vi "MRC Ds Comms Wait For System Server.vi"(8 "error in (no error)":errorcluster, 11 "waitTimeMs":u32) -> (0 "error out":errorcluster)   [LabVIEW 2026, in "MrcLib.lvlib"]
doc: "MRC_Bool MRC_CALLCONV MRC_DsComms_WaitForSystemServer(uint32_t waitTimeMs);"
uses:
  MrcLib.lvlib
  MrcLib.dll
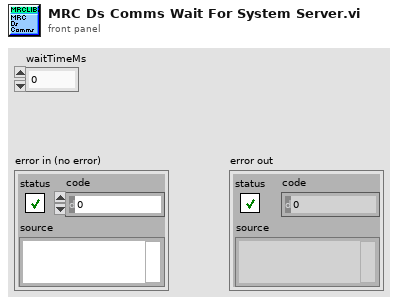
[diagram p1: front panel]
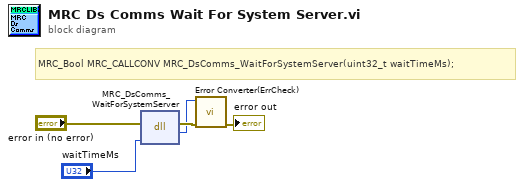
[diagram p0: block diagram]
diagram:
  # "MRC_Bool MRC_CALLCONV MRC_DsComms_WaitForSystemServer(uint32_t waitTimeMs);"
  n1 = dll-call lib="MrcLib.*" fn="MRC_DsComms_WaitForSystemServer"(error in="error in (no error)", "waitTimeMs"="waitTimeMs") -> (error out=w3:errorcluster, "return type"=w1:u8)  [unwired: 3 in, 1 out]
  n2 = call <vilib>:"Error Converter(ErrCheck).vi"("error in (no error)"=w3, "status"=w1) -> ("error out"=→"error out":errorcluster)  [unwired: 9 in]
